vi "Draw Single Icon Core.vi"(4 "Background Color":u32(colorbox), 5 "Mouse State":T1, 6 "Icon Size":T3, 7 "Border Size":i16, 8 "error in (no error)":errorcluster, 9 "Image Path":path, 10 "Image Data":T2, 11 "Toolbar Control in":refnum<class "Toolbar Control.lvclass">) -> (0 "error out":errorcluster, 2 "Icon Image Out":T2, 3 "Toolbar Control out":refnum<class "Toolbar Control.lvclass">)   [LabVIEW 2011, in "Toolbar Control.lvclass"]
doc: "This VI will create the image provided by either <B>Image Data</B> or <B>Image Path</B> and return the <B>Icon Image Out</B> which resizes the image, adds background, and then overlays for Mouse Over and Mouse Down provided by <B>Mouse State</B> and <B>Background Color</B>.\n\n-------------\nDeveloped by Brian Hoover (hooovahh)"
uses:
  Toolbar Control.lvclass
  <vilib>/picture/picture.llb/imagedata.ctl
  <vilib>/Utility/miscctls.llb/LVBoundsTypeDef.ctl
  Controls/Mouse State.ctl
  Toolbar Control.lvclass/Toolbar Control.ctl
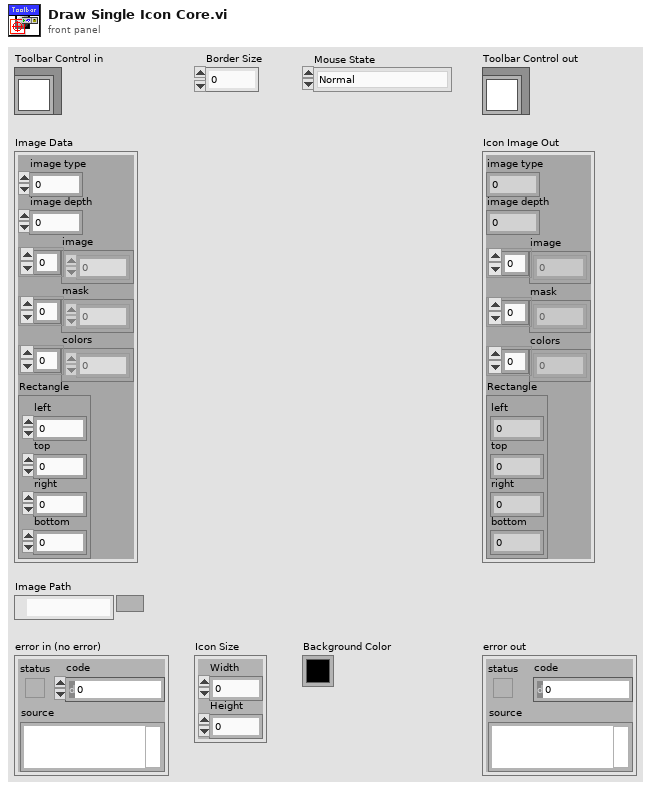
[diagram p1: front panel]
types:
  T1 = typedef "Mouse State.ctl" = enum8{"Normal", "Mouse Over", "Mouse Down"}
  T2 = typedef "imagedata.ctl" = cluster{"image type":i32, "image depth":i32, "image":u8[], "mask":u8[], "colors":u32[], "Rectangle":cluster{"left":i16, "top":i16, "right":i16, "bottom":i16}}
  T3 = typedef "LVBoundsTypeDef.ctl" = cluster{"Width":u32, "Height":u32}
  T4 = cluster{"left":i16, "top":i16, "right":i16, "bottom":i16}
  T5 = typedef "LVRectTypeDef.ctl" = cluster{"Left":i16, "Top":i16, "Right":i16, "Bottom":i16}
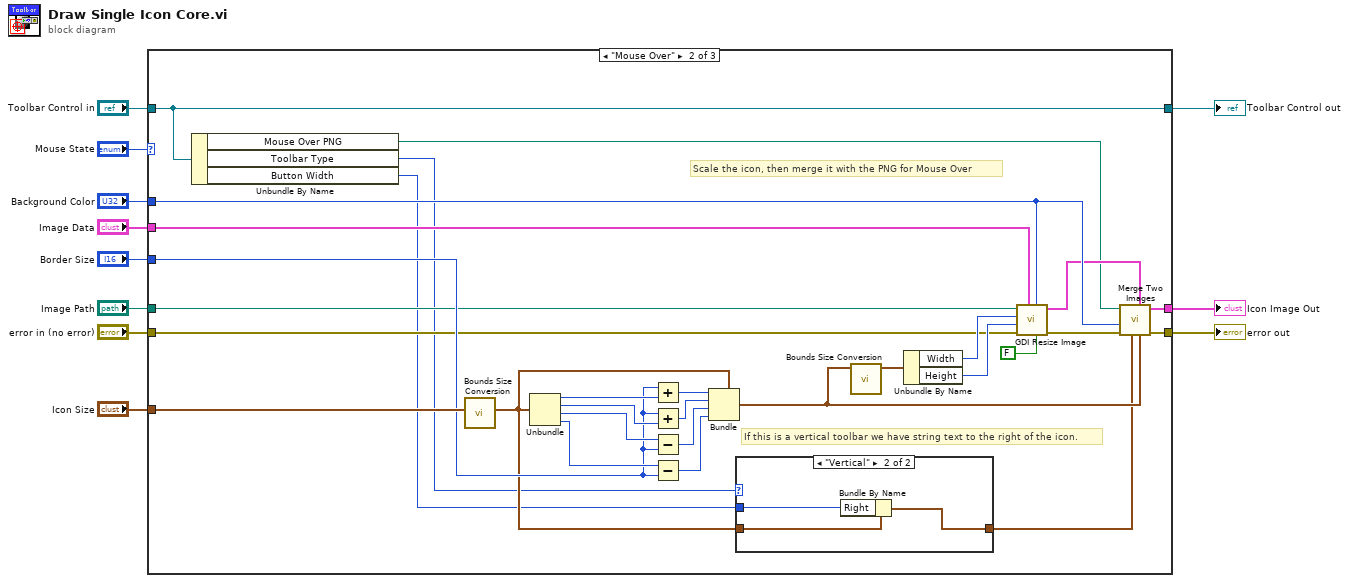
[diagram p0: block diagram]
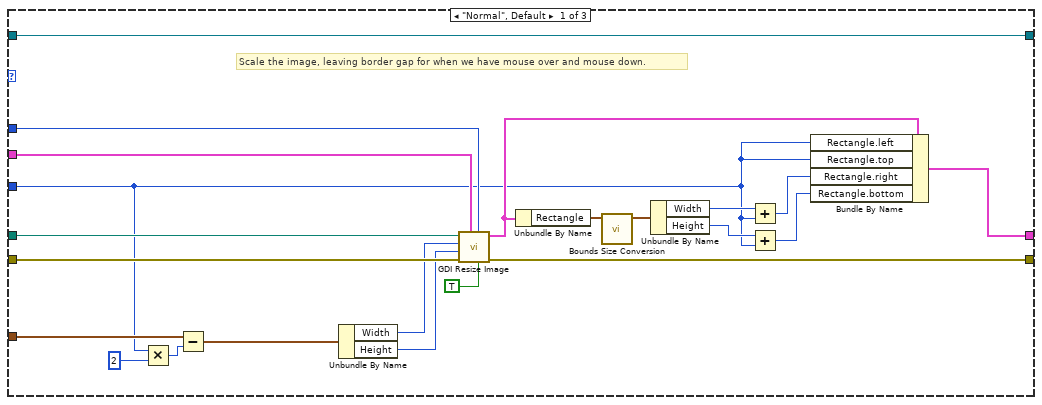
[diagram p2: hidden frame]
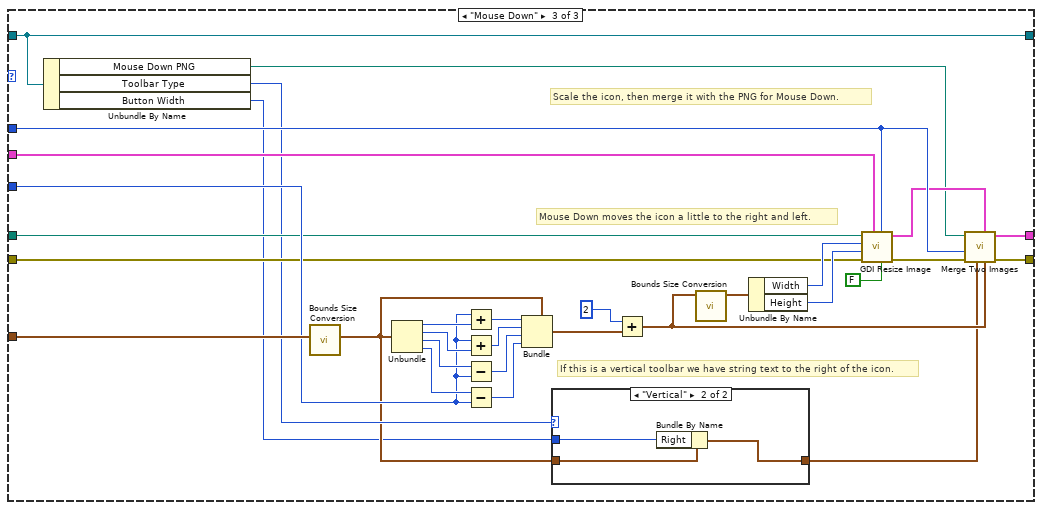
[diagram p4: hidden frame]
diagram:
  n1 = case shown="\"Mouse Over\"" "Mouse State" {
    tunnel: [w33 w42 w77] -> w11
    tunnel: "error in (no error)" -> [w32 w44 w79]
    tunnel: [w31 w41 w76] -> w9
    tunnel: "Border Size" -> [w15 w53 w88]
    tunnel: "Icon Size" -> [w21 w62 w97]
    tunnel: "Background Color" -> [w20 w49 w84]
    tunnel: "Image Data" -> [w19 w50 w85]
    tunnel: "Image Path" -> [w18 w51 w86]
    tunnel: "Toolbar Control in" -> [w12 w37 w72]
    tunnel: [w12 w37 w72] -> w1
    frame "Normal", Default {
      # "Scale the image, leaving border gap for when we have mouse over and mouse down."
      n2 = Multiply(x=w15, y=i16 2) -> (x*y=w14:i16)
      n3 = Subtract(x=w21, y=w14) -> (x-y=w16:T3)
      n4 = Unbundle By Name(w16) -> ("Width"=w22:u32, "Height"=w23:u32)
      n5 = call "GDI Resize Image.vi"("Set Background Color (T)"=TRUE, "Background Color"=w20, "Image Data"=w19, "error in (no error)"=w32, "Height"=w23, "Width"=w22, "Path"=w18) -> ("error out"=w31:errorcluster, "Resized image data"=w30:T2)  [unwired: 3 in]
      n6 = Unbundle By Name(w30) -> ("Rectangle"=w29:T4)
      n7 = call "Bounds Size Conversion.vi"("Bounds"=w29) -> ("Size Out"=w28:T3)  [unwired: 9 in, 1 out]
      n8 = Unbundle By Name(w28) -> ("Width"=w27:u32, "Height"=w25:u32)
      n9 = Add(x=w27, y=w15) -> (x+y=w26:u32)
      n10 = Add(x=w25, y=w15) -> (x+y=w24:u32)
      n11 = Bundle By Name(cluster=w30, "Rectangle.left"=w15, "Rectangle.top"=w15, "Rectangle.right"=w26, "Rectangle.bottom"=w24) -> (w33:T2)
    }
    frame "Mouse Over" {
      # "Scale the icon, then merge it with the PNG for Mouse Over"
      # "If this is a vertical toolbar we have string text to the right of the icon."
      n12 = Unbundle By Name(w37) -> ("Mouse Over PNG"=w36:path, "Toolbar Type"=w35:enum16{"Horizontal", "Vertical"}, "Button Width"=w34:i32)
      n13 = call "Bounds Size Conversion.vi"("Size"=w62) -> ("Bounds Out"=w39:T5)  [unwired: 9 in, 1 out]
      n14 = Unbundle(w39) -> ("Left"=w61:i16, "Top"=w60:i16, "Right"=w59:i16, "Bottom"=w58:i16)
      n15 = Add(x=w53, y=w61) -> (x+y=w57:i16)
      n16 = Add(x=w53, y=w60) -> (x+y=w56:i16)
      n17 = Subtract(x=w59, y=w53) -> (x-y=w55:i16)
      n18 = Subtract(x=w58, y=w53) -> (x-y=w54:i16)
      n19 = Bundle(cluster=w39, "Left"=w57, "Top"=w56, "Right"=w55, "Bottom"=w54) -> (w48:T5)
      n20 = case shown="\"Vertical\"" w35 {
        tunnel: w39 -> [w63 w66]
        tunnel: [w63 w65] -> w38
        tunnel: w34 -> [_ w64]
        frame "Horizontal", Default {
        }
        frame "Vertical" {
          n21 = Bundle By Name(cluster=w66, "Right"=w64) -> (w65:T5)
        }
      }
      n22 = call "Bounds Size Conversion.vi"("Bounds"=w48) -> ("Size Out"=w47:T3)  [unwired: 9 in, 1 out]
      n23 = Unbundle By Name(w47) -> ("Width"=w46:u32, "Height"=w45:u32)
      n24 = call "GDI Resize Image.vi"("Set Background Color (T)"=FALSE ("Set Background Color? (T)"), "Background Color"=w49, "Image Data"=w50, "error in (no error)"=w44, "Height"=w45, "Width"=w46, "Path"=w51) -> ("error out"=w43:errorcluster, "Resized image data"=w40:T2)  [unwired: 3 in]
      n25 = call "Merge Two Images.vi"("Image 2 Bounds"=w48, "Image 2 Data"=w40, "Image 1 Bounds"=w38, "error in (no error)"=w43, "Background Color"=w49, "Image 1 Path"=w36) -> ("error out"=w41:errorcluster, "Merged Image Data"=w42:T2)  [unwired: 4 in]
    }
    frame "Mouse Down" {
      # "Scale the icon, then merge it with the PNG for Mouse Down."
      # "Mouse Down moves the icon a little to the right and left."
      # "If this is a vertical toolbar we have string text to the right of the icon."
      n26 = Unbundle By Name(w72) -> ("Mouse Down PNG"=w71:path, "Toolbar Type"=w70:enum16{"Horizontal", "Vertical"}, "Button Width"=w67:i32)
      n27 = call "Bounds Size Conversion.vi"("Size"=w97) -> ("Bounds Out"=w69:T5)  [unwired: 9 in, 1 out]
      n28 = Unbundle(w69) -> ("Left"=w96:i16, "Top"=w95:i16, "Right"=w94:i16, "Bottom"=w93:i16)
      n29 = Add(x=w88, y=w96) -> (x+y=w92:i16)
      n30 = Add(x=w88, y=w95) -> (x+y=w91:i16)
      n31 = Subtract(x=w94, y=w88) -> (x-y=w90:i16)
      n32 = Subtract(x=w93, y=w88) -> (x-y=w89:i16)
      n33 = Bundle(cluster=w69, "Left"=w92, "Top"=w91, "Right"=w90, "Bottom"=w89) -> (w83:T5)
      n34 = case shown="\"Vertical\"" w70 {
        tunnel: w69 -> [w98 w101]
        tunnel: [w98 w100] -> w68
        tunnel: w67 -> [_ w99]
        frame "Horizontal", Default {
        }
        frame "Vertical" {
          n35 = Bundle By Name(cluster=w101, "Right"=w99) -> (w100:T5)
        }
      }
      n36 = Add(x=i16 2 ("Border Size 2"), y=w83) -> (x+y=w74:T5)
      n37 = call "Bounds Size Conversion.vi"("Bounds"=w74) -> ("Size Out"=w82:T3)  [unwired: 9 in, 1 out]
      n38 = Unbundle By Name(w82) -> ("Width"=w81:u32, "Height"=w80:u32)
      n39 = call "GDI Resize Image.vi"("Set Background Color (T)"=FALSE ("Set Background Color? (T)"), "Background Color"=w84, "Image Data"=w85, "error in (no error)"=w79, "Height"=w80, "Width"=w81, "Path"=w86) -> ("error out"=w78:errorcluster, "Resized image data"=w75:T2)  [unwired: 3 in]
      n40 = call "Merge Two Images.vi"("Image 2 Bounds"=w74, "Image 2 Data"=w75, "Image 1 Bounds"=w68, "error in (no error)"=w78, "Background Color"=w84, "Image 1 Path"=w71) -> ("error out"=w76:errorcluster, "Merged Image Data"=w77:T2)  [unwired: 4 in]
    }
  }
  "Icon Image Out" <- w11
  "error out" <- w9
  "Toolbar Control out" <- w1
